vi "Climb_Globals.vi"() -> ()   [LabVIEW 2018]
uses:
  Subsytems/Climb/Climb_Notifier.ctl
  Subsytems/Climb/Climb_Control_Type.ctl
panel:
  in  "Climb_Servo_Two":string="Climb_Servo_Two"
  in  "Climb_Servo":string="Climb_Servo"
  out "Climb_Extended":bool
  out "Climb_Retracted":bool
  in  "Climb_IR_Rear":string="Climb_IR_Rear"
  out "Distance_Hit":bool
  in  "Intake_IR":string="Intake_IR"
  in  "Climb_IR":string="Climb_IR"
  in  "Bottom_Climb_Limit_Back":string="Bottom_Climb_Limit_Back"
  in  "Top_Climb_Limit_Back":string="Top_Climb_Limit_Back"
  in  "Back_Brake":string="Back_Brake"
  in  "Back_Elevator_Slave":string="Back_Elevator_Slave"
  in  "Back_Elevator_Master":string="Back_Elevator_Master"
  in  "Climb_Execute_Notifier_Ref":refnum<notifier>
  in  "Climb_Set_Notifier_Ref":refnum<notifier>
  in  "Climb_Execute_Notifier":string="Climb_Execute_Notifier"
  in  "Climb_Set_Notifier":string="Climb_Set_Notifier"
  in  "Right_Drive":string="Right_Drive"
  in  "Left_Drive":string="Left_Drive"
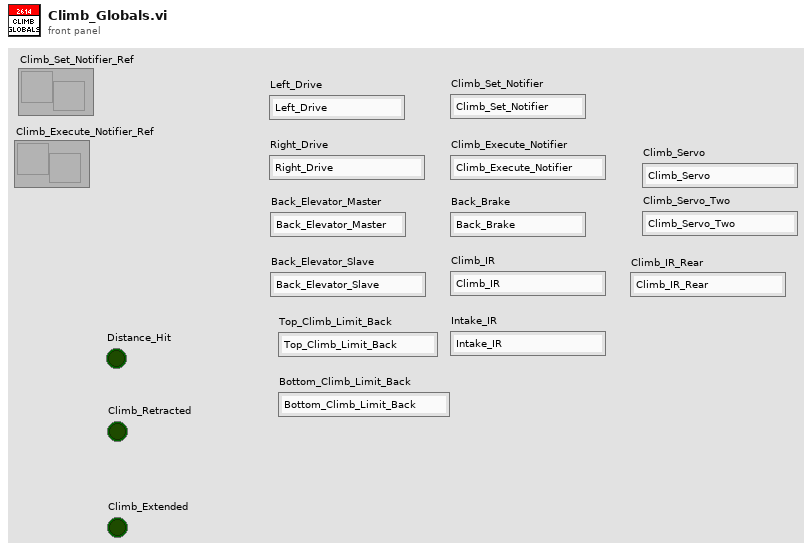
[diagram p1: front panel]
diagram:
